vi "ScanNumToFilePath.vi"(4 "# Elements":i32=5, 5 "Additional Axis?":bool, 6 "Dig Config":i32, 7 "Full Array Scan?":bool, 8 "Scan to View":u32, 9 "number of scan planes":i32=1, 10 "Synth App?":bool, 11 "Root File Name":string) -> (0 "String":string, 1 "error out":errorcluster, 3 "appended path":path)   [LabVIEW 2022 SP3]
uses:
  Motion Controllers/-MotionRoutines/MotionGlobals.vi
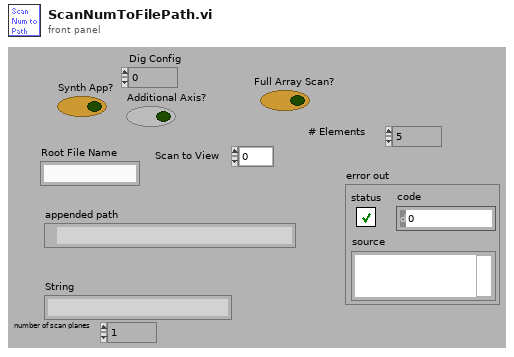
[diagram p1: front panel]
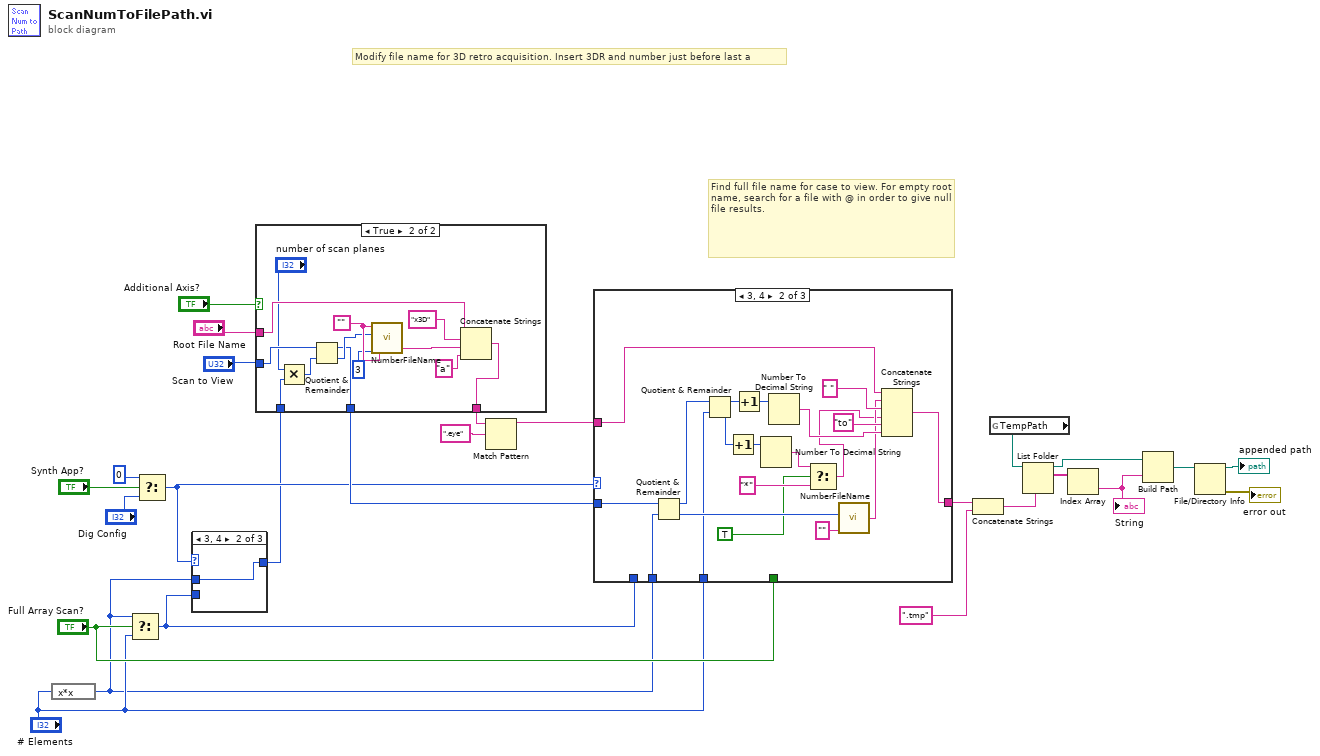
[diagram p0: block diagram]
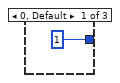
[diagram p2: hidden frame]
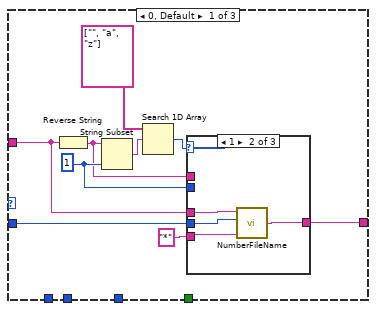
[diagram p5: hidden frame]
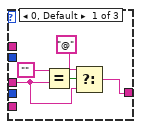
[diagram p6: hidden frame]
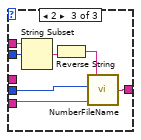
[diagram p7: hidden frame]
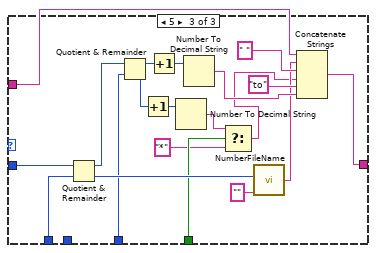
[diagram p8: hidden frame]
diagram:
  # "Modify file name for 3D retro acquisition. Insert 3DR and number just before last a"
  # "Find full file name for case to view. For empty root name, search for a file with @ in order to give null file results."
  n1 = expression code="x*x"("# Elements") -> (w1:i32)
  n2 = Select(t=w1, s="Full Array Scan?", f="# Elements") -> (s? t:f=w5:i32)
  n3 = Select(t=0, s="Synth App?", f="Dig Config") -> (s? t:f=w7:i32)
  n4 = case shown="3, 4" w7 {
    tunnel: [1 w28 w29] -> w6
    tunnel: w5 -> [_ _ w29]
    tunnel: w1 -> [_ w28 _]
    frame 0, Default {
    }
    frame 3, 4 {
    }
    frame 5 {
    }
  }
  n5 = case shown="True" "Additional Axis?" {
    tunnel: [w31 w39] -> w11
    tunnel: "Root File Name" -> [w31 w36]
    tunnel: "Scan to View" -> [w30 w34]
    tunnel: [w30 w37] -> w8
    tunnel: w6 -> [_ w35]
    frame False {
    }
    frame True {
      w41 = ""
      n6 = Multiply(x="number of scan planes", y=w35) -> (x*y=w33:i32)
      n7 = Quotient & Remainder(x=w34, y=w33) -> (x-y*floor(x/y)=w37:u32, floor(x/y)=w38:u32)
      n8 = call "NumberFileName.vi"("String"=w41, "Digits"=3, "File number"=w38, "file name"=w41) -> ("Numbered File"=w43:string)
      n9 = Concatenate Strings(w36, "x3D" ("string"), w43, "a" ("string")) -> (w39:string)
    }
  }
  n10 = Match Pattern(string=w11, regular expression=".eye") -> (before substring=w20:string)  [unwired: 4 out]
  n11 = case shown="3, 4" w7 {
    tunnel: [w48 w79 w99] -> w22
    tunnel: w20 -> [w47 w77 w97]
    tunnel: w8 -> [w46 w89 w109]
    tunnel: w5 -> [_ _ w96]
    tunnel: "Full Array Scan?" -> [_ _ w95]
    tunnel: "# Elements" -> [_ w71 w90]
    tunnel: w1 -> [_ w70 _]
    frame 0, Default {
      w53 = 1
      n12 = Reverse String(1:w47) -> (0:w52:string)
      n13 = String Subset(string=w52, length (rest)=w53) -> (substring=w50:string)  [unwired: 1 out]
      n14 = Search 1D Array(1D array=string[] ["", "a", "z"] ("Array"), element=w50) -> (index of element=w51:i32)  [unwired: 1 out]
      n15 = case shown="1" w51 {
        tunnel: w46 -> [_ w62 w69]
        tunnel: w47 -> [w56 w59 _]
        tunnel: "*" -> [_ w60 w67]
        tunnel: [w54 w61 w68] -> w48
        tunnel: w52 -> [_ _ w64]
        tunnel: w53 -> [_ _ w63]
        frame 0, Default {
          n16 = Equal?(x="", y=w56) -> (x = y?=w57:bool)
          n17 = Select(t="@", s=w57, f=w56) -> (s? t:f=w54:string)
        }
        frame 1 {
          n18 = call "NumberFileName.vi"("String"=w60, "File number"=w62, "file name"=w59) -> ("Numbered File"=w61:string)  [unwired: 1 in]
        }
        frame 2 {
          n19 = String Subset(string=w64, offset (0)=w63) -> (substring=w65:string)  [unwired: 1 out]
          n20 = Reverse String(1:w65) -> (0:w66:string)
          n21 = call "NumberFileName.vi"("String"=w67, "File number"=w69, "file name"=w66) -> ("Numbered File"=w68:string)  [unwired: 1 in]
        }
      }
    }
    frame 3, 4 {
      n22 = Quotient & Remainder(x=w89, y=w70) -> (x-y*floor(x/y)=w87:u32, floor(x/y)=w88:u32)
      n23 = Quotient & Remainder(x=w87, y=w71) -> (x-y*floor(x/y)=w86:u32, floor(x/y)=w85:u32)
      n24 = Increment(x=w85) -> (x+1=w84:u32)
      n25 = Increment(x=w86) -> (x+1=w83:u32)
      n26 = Number To Decimal String(number=w84) -> (decimal integer string=w76:string)  [unwired: 1 out]
      n27 = Number To Decimal String(number=w83) -> (decimal integer string=w80:string)  [unwired: 1 out]
      n28 = Select(t=w76, s=TRUE ("Full Array Scan?"), f="*") -> (s? t:f=w75:string)
      n29 = call "NumberFileName.vi"("String"="", "File number"=w88) -> ("Numbered File"=w78:string)  [unwired: 2 in]
      n30 = Concatenate Strings(w77, w78, " ", w75, "to", w80) -> (w79:string)
    }
    frame 5 {
      n31 = Quotient & Remainder(x=w109, y=w96) -> (x-y*floor(x/y)=w107:u32, floor(x/y)=w108:u32)
      n32 = Quotient & Remainder(x=w107, y=w90) -> (x-y*floor(x/y)=w106:u32, floor(x/y)=w105:u32)
      n33 = Increment(x=w105) -> (x+1=w104:u32)
      n34 = Increment(x=w106) -> (x+1=w103:u32)
      n35 = Number To Decimal String(number=w104) -> (decimal integer string=w94:string)  [unwired: 1 out]
      n36 = Number To Decimal String(number=w103) -> (decimal integer string=w100:string)  [unwired: 1 out]
      n37 = Select(t=w94, s=w95, f="*") -> (s? t:f=w93:string)
      n38 = call "NumberFileName.vi"("String"="", "File number"=w108) -> ("Numbered File"=w98:string)  [unwired: 2 in]
      n39 = Concatenate Strings(w97, w98, " ", w93, "to", w100) -> (w99:string)
    }
  }
  n40 = Concatenate Strings(w22, ".tmp") -> (w21:string)
  n41 = global read "MotionGlobals.vi" "TempPath"() -> (w12:path)
  n42 = List Folder(path=w12, pattern=w21) -> (path out=w24:path, filenames=w23:string[])  [unwired: 1 in, 3 out]
  n43 = Index Array(array=w23) -> (element=w26:string)  [unwired: 1 in]
  "String" <- w26
  n44 = Build Path(base path=w24, name or relative path=w26) -> (appended path=w19:path)
  n45 = File/Directory Info(path=w19) -> (path out=→"appended path":path, error out=→"error out":errorcluster)  [unwired: 1 in, 5 out]
